vi "tmp_arduino_parser.vi"() -> ()   [LabVIEW 2018]
uses:
  <vilib>/xml/NI_XML.lvlib
panel:
  out "Valves":dbl[][](array[numeric])
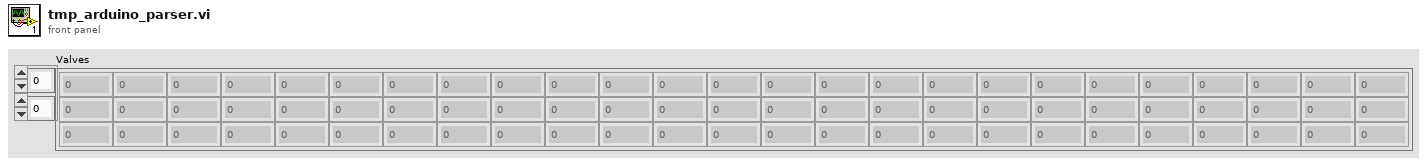
[diagram p1: front panel]
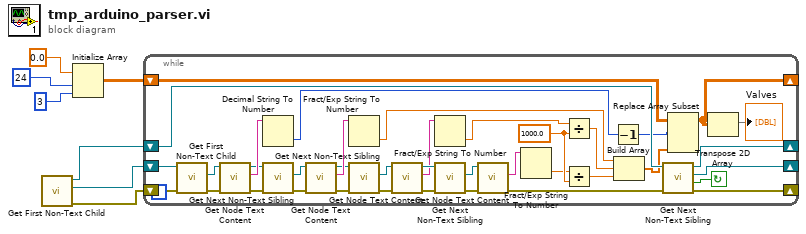
[diagram p0: block diagram]
diagram:
  n1 = call <vilib>:"Get First Non-Text Child.vi"() -> ("error out"=w4:errorcluster, "child node"=w5:refnum<k20>, "node out"=w1:refnum<k20>, "error in (no error)"=w6:errorcluster, "node in"=w7:refnum<k20>)  [unwired: 6 in, 1 out]
  n2 = Initialize Array(0.0, 24, 3 ("dimension size")) -> (w2:dbl[][])
  n3 = while {
    shift-right: [w41] -> _
    shift-left: w4 -> [w23]
    shift-right: [w42] -> _
    shift-left: w5 -> [w24]
    shift-right: [w12] -> _
    shift-left: w2 -> [w15]
    shift-right: [w21] -> _
    shift-left: w1 -> [w22]
    stop <- w40 continue-if-true
    w20 = 1000.0
    n4 = call <vilib>:"Get First Non-Text Child.vi"("error in (no error)"=w23, "node in"=w24) -> ("error out"=w26:errorcluster, "child node"=w25:refnum<k20>)  [unwired: 6 in, 2 out]
    n5 = call <vilib>:"Get Node Text Content.vi"("error in (no error)"=w26, "node in"=w25) -> ("error out"=w43:errorcluster, "node text"=w46:string, "node out"=w44:refnum<k20>)  [unwired: 7 in]
    n6 = Decimal String To Number(string=w46) -> (number=w38:i32)  [unwired: 2 in, 1 out]
    n7 = call <vilib>:"Get Next Non-Text Sibling.vi"("error in (no error)"=w43, "node in"=w44) -> ("error out"=w45:errorcluster, "sibling node"=w39:refnum<k20>)  [unwired: 6 in, 2 out]
    n8 = call <vilib>:"Get Node Text Content.vi"("error in (no error)"=w45, "node in"=w39) -> ("error out"=w34:errorcluster, "node text"=w47:string, "node out"=w35:refnum<k20>)  [unwired: 7 in]
    n9 = Fract/Exp String To Number(string=w47) -> (number=w10:dbl)  [unwired: 3 in, 1 out]
    n10 = call <vilib>:"Get Next Non-Text Sibling.vi"("error in (no error)"=w34, "node in"=w35) -> ("error out"=w37:errorcluster, "sibling node"=w36:refnum<k20>)  [unwired: 6 in, 2 out]
    n11 = call <vilib>:"Get Node Text Content.vi"("error in (no error)"=w37, "node in"=w36) -> ("error out"=w29:errorcluster, "node text"=w28:string, "node out"=w30:refnum<k20>)  [unwired: 7 in]
    n12 = Fract/Exp String To Number(string=w28) -> (number=w18:dbl)  [unwired: 3 in, 1 out]
    n13 = call <vilib>:"Get Next Non-Text Sibling.vi"("error in (no error)"=w29, "node in"=w30) -> ("error out"=w33:errorcluster, "sibling node"=w32:refnum<k20>)  [unwired: 6 in, 2 out]
    n14 = call <vilib>:"Get Node Text Content.vi"("error in (no error)"=w33, "node in"=w32) -> ("error out"=w31:errorcluster, "node text"=w27:string)  [unwired: 7 in, 1 out]
    n15 = Fract/Exp String To Number(string=w27) -> (number=w19:dbl)  [unwired: 3 in, 1 out]
    n16 = Divide(x=w18, y=w20) -> (x/y=w17:dbl)
    n17 = Divide(x=w19, y=w20) -> (x/y=w16:dbl)
    n18 = Decrement(x=w38) -> (x-1=w14:i32)
    n19 = Build Array(w10, w17, w16) -> (w13:dbl[])
    n20 = call <vilib>:"Get Next Non-Text Sibling.vi"("error in (no error)"=w31, "node in"=w22) -> ("error out"=w41:errorcluster, "found sibling node?"=w40:bool, "sibling node"=w42:refnum<k20>, "node out"=w21:refnum<k20>)  [unwired: 6 in]
    n21 = Replace Array Subset(array=w15, new element=w13, index (row)=w14) -> (w12:dbl[][])  [unwired: 1 in]
    n22 = Transpose 2D Array(2D array=w12) -> (transposed array=→"Valves":dbl[][])
  }
